vi "compare channel list to typedefs.vi"(8 "error in":errorcluster, 11 "configured channels in":refnum<class "TBM channel.lvclass">[](array[class])) -> (0 "error out":errorcluster, 3 "configured channels out":refnum<class "TBM channel.lvclass">[](array[class]))   [LabVIEW 2013, in "fixed channel tag bus module configuration.lvclass"]
uses:
  fixed channel tag bus module configuration.lvclass
  <vilib>/NI/Tag Bus Module Framework/channel/TBM channel.lvclass
  <vilib>/NI/Tag Bus/tag/tag descriptor.lvclass/tag descriptor.ctl
  <vilib>/NI/Tag Bus/tag/tag descriptor.lvclass
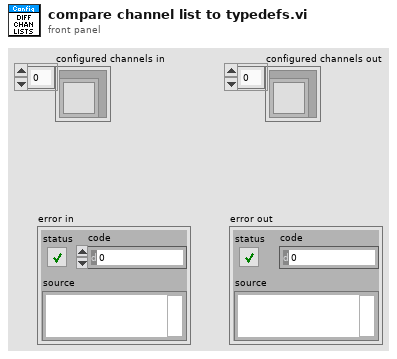
[diagram p1: front panel]
types:
  T1 = typedef "tag bus.lvlib/tag descriptor.lvclass/Data Type.ctl" = enum16{"Double", "Single", "I64", "I32", "I16", "I8", "U64", "U32", "U16", "U8", "Boolean", "String", "Array of Double", "Array of Single", "Array of I64", "Array of I32", "Array of I16", "Array of I8", "Array of U64", "Array of U32", "Array of U16", "Array of U8", "Array of Boolean", "Array of String"}
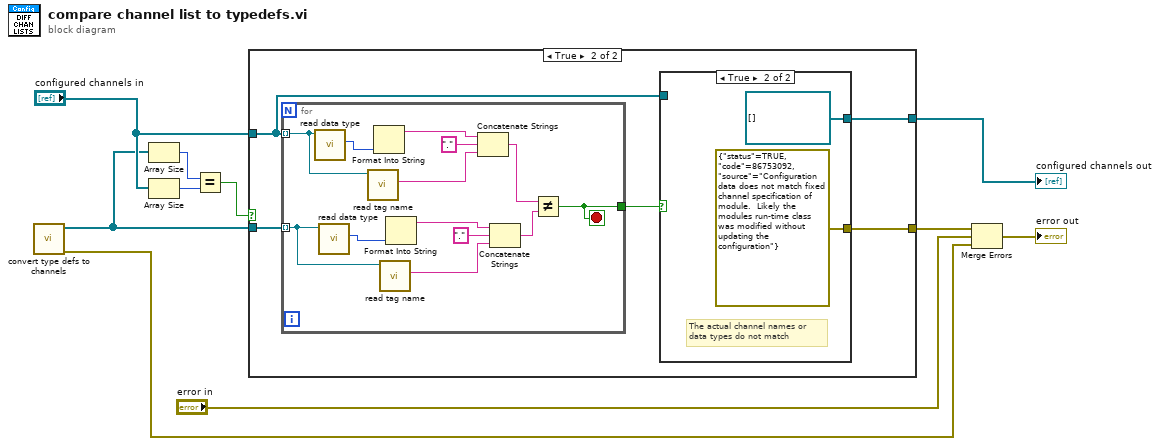
[diagram p0: block diagram]
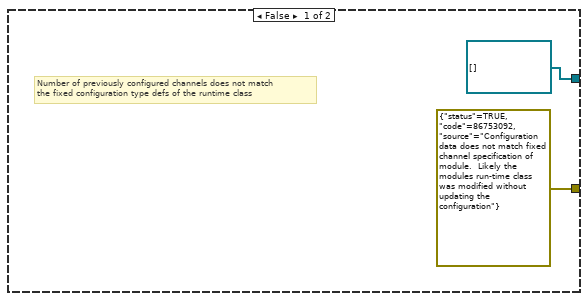
[diagram p2: hidden frame]
diagram:
  n1 = call "convert type defs to channels.vi"() -> ("error out"=w1:errorcluster, "Array out"=w2:refnum<class "TBM channel.lvclass">[])  [unwired: 10 in]
  n2 = Array Size(array=w2) -> (size(s)=w8:i32)
  n3 = Array Size(array="configured channels in") -> (size(s)=w7:i32)
  n4 = Equal?(x=w8, y=w7) -> (x = y?=w5:bool)
  n5 = case shown="True" w5 {
    tunnel: "configured channels in" -> [_ w15]
    tunnel: [errorcluster {"status"=TRUE, "code"=86753092, "source"="Configuration data does not match fixed channel specification of module.  Likely the modules run-time class was modified without updating the configuration"} ("error constant") w16] -> w9
    tunnel: [refnum<class "TBM channel.lvclass">[] [] ("configured channels") w14] -> w10
    tunnel: w2 -> [_ w13]
    frame False {
      # "Number of previously configured channels does not match\nthe fixed configuration type defs of the runtime class"
    }
    frame True {
      n6 = for {
        tunnel: w15 -> [w30] mode=indexing
        tunnel: [w29] -> w17
        tunnel: w13 -> [w22] mode=indexing
        stop <- w29 stop-if-true
        n7 = call <vilib>:"read data type.vi"("system tag in"=w30) -> ("data type"=w33:T1)  [unwired: 8 in, 2 out]
        n8 = call <vilib>:"read data type.vi"("system tag in"=w22) -> ("data type"=w23:T1)  [unwired: 8 in, 2 out]
        n9 = call <vilib>:"read tag name.vi"("system tag in"=w30) -> ("name"=w32:string)  [unwired: 8 in, 2 out]
        n10 = Format Into String(w33) -> (resulting string=w31:string)  [unwired: 3 in, 1 out]
        n11 = call <vilib>:"read tag name.vi"("system tag in"=w22) -> ("name"=w24:string)  [unwired: 8 in, 2 out]
        n12 = Format Into String(w23) -> (resulting string=w25:string)  [unwired: 3 in, 1 out]
        n13 = Concatenate Strings(w31, "." ("resulting string"), w32) -> (w27:string)
        n14 = Concatenate Strings(w25, "." ("resulting string"), w24) -> (w21:string)
        n15 = Not Equal?(x=w27, y=w21) -> (x != y?=w29:bool)
      }
      n16 = case shown="True" w17 {
        tunnel: [_ errorcluster {"status"=TRUE, "code"=86753092, "source"="Configuration data does not match fixed channel specification of module.  Likely the modules run-time class was modified without updating the configuration"} ("error constant")] -> w16
        tunnel: w15 -> [w18 _]
        tunnel: [w18 refnum<class "TBM channel.lvclass">[] [] ("configured channels")] -> w14
        frame False {
        }
        frame True {
          # "The actual channel names or\ndata types do not match"
        }
      }
    }
  }
  "configured channels out" <- w10
  n17 = Merge Errors(w9, "error in", w1) -> (→"error out":errorcluster)
